vi "Anti_Reset_Windup.vi"(2 "Integrator enabled range":dbl=0.02 min=0.0 max=0.1 step=0.01, 3 "Ti_enabled_in":dbl, 4 "actuall error":dbl) -> (1 "Ti_out":dbl)   [LabVIEW 2013]
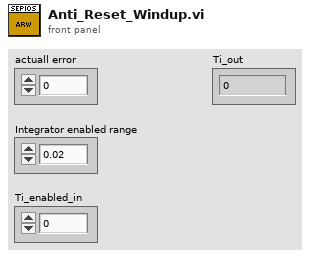
[diagram p1: front panel]
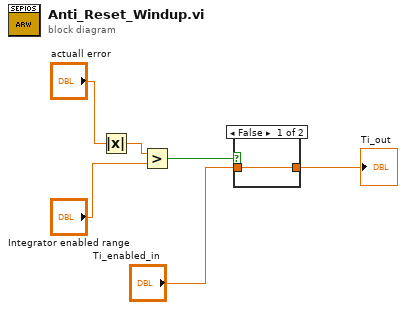
[diagram p0: block diagram]
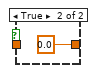
[diagram p2: hidden frame]
diagram:
  n1 = Absolute Value(x="actuall error") -> (abs(x)=w2:dbl)
  n2 = Greater?(x=w2, y="Integrator enabled range") -> (0:w4:bool)
  n3 = case shown="False" w4 {
    tunnel: [w7 0.0] -> w5
    tunnel: "Ti_enabled_in" -> [w7 _]
    frame False {
    }
    frame True {
    }
  }
  "Ti_out" <- w5
